vi "Modbus.Disconnect.vi"(8 "error in (no error)":errorcluster) -> (0 "error out":errorcluster)   [LabVIEW 2019, in "Modbus.lvlib"]
uses:
  Modbus.lvlib
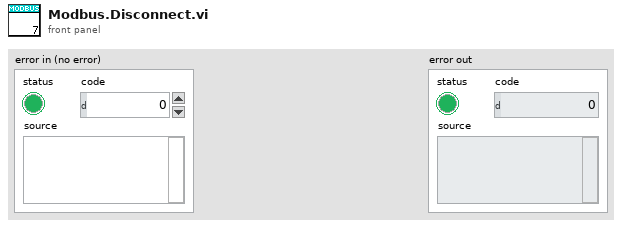
[diagram p1: front panel]
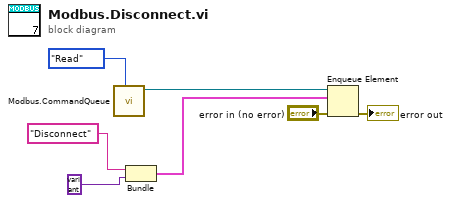
[diagram p0: block diagram]
diagram:
  n1 = call "Modbus.CommandQueue.vi"("OP"=enum16{"Read", "Write"}."Read") -> ("queue OUT"=w6:refnum<queue>)  [unwired: 10 in]
  n2 = Bundle("Disconnect", variant) -> (w4:cluster{string, variant})  [unwired: 1 in]
  n3 = Enqueue Element(queue=w6, element=w4, error in (no error)="error in (no error)") -> (error out=→"error out":errorcluster)  [unwired: 1 in, 2 out]
